vi "SysLog cRIO store messages.vi"(8 "Fehler (in)":errorcluster caption="Fehlerkonstante") -> (0 "Fehler (out)":errorcluster caption="Fehlerkonstante")   [LabVIEW 2020, in "SysLog_cRIO.lvlib"]
doc: "ErrorLogHistory cRIO - Meldungen speichern\nappand to log file - along with BSZ\n\nriw - 11.06.2018"
uses:
  SysLog_cRIO.lvlib
  Allgemein/allgemeine Sub-VIs.lvlib
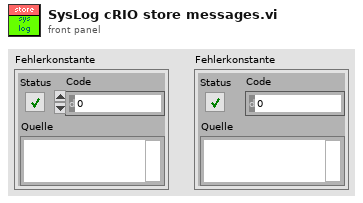
[diagram p1: front panel]
types:
  T1 = enum16{"open", "replace", "create", "open or create", "replace or create", "replace or create with confirmation"}
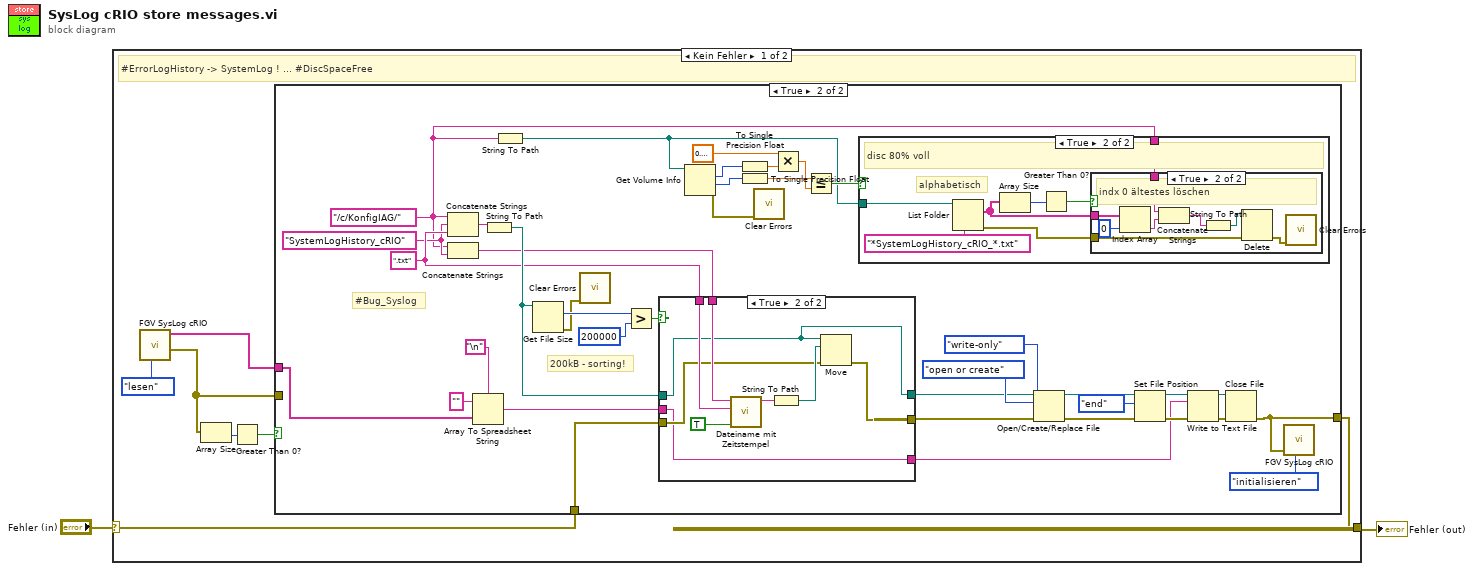
[diagram p0: block diagram]
diagram:
  n1 = case shown="Kein Fehler" "Fehler (in)" {
    selector: "Fehler (in)" -> [w6 w75]
    tunnel: [w5 w75] -> w2
    frame No Error {
      # "#ErrorLogHistory -> SystemLog ! ... #DiscSpaceFree"
      n2 = call "FGV SysLog cRIO.vi"("Aktion"=enum16{"initialisieren", "lesen", "schreiben"}."lesen") -> ("Fehler Array  out"=w3:errorcluster[], "Message out"=w7:string[])  [unwired: 8 in, 1 out]
      n3 = Array Size(array=w3) -> (size(s)=w8:i32)
      n4 = Greater Than 0?(x=w8) -> (x > 0?=w4:bool)
      n5 = case shown="True" w4 {
        tunnel: w7 -> [_ w13]
        tunnel: w3 -> [_ _]
        tunnel: w6 -> [_ w45]
        tunnel: [_ w23] -> w5
        frame False {
        }
        frame True {
          w10 = "/c/KonfigIAG/" ("String")
          w38 = ".txt" ("String")
          w11 = "SystemLogHistory_cRIO" ("String")
          # "#Bug_Syslog"
          # "200kB - sorting!"
          n6 = Concatenate Strings(w10, w11, w38) -> (w40:string)
          n7 = Concatenate Strings(w10, w11) -> (w12:string)
          n8 = Array To Spreadsheet String(delimiter (Tab)="\n", array=w13, 3:"" ("Format-String")) -> (spreadsheet string=w46:string)
          n9 = String To Path(string=w40) -> (path=w39:path)
          n10 = String To Path(string=w10) -> (path=w14:path)
          n11 = Get File Size(file=w39) -> (size (in bytes)=w43:i64, 0:w42:errorcluster)  [unwired: 1 in, 1 out]
          n12 = call <vilib>:"Clear Errors.vi"("error in (no error)"=w42) -> ()  [unwired: 5 in, 2 out]
          n13 = Greater?(x=w43, y=i64 200000) -> (0:w41:bool)
          n14 = case shown="True" w41 {
            tunnel: w46 -> [w64 w66]
            tunnel: w39 -> [w65 w67]
            tunnel: w45 -> [w63 w69]
            tunnel: w12 -> [_ w73]
            tunnel: w38 -> [_ w72]
            tunnel: [w63 w68] -> w27
            tunnel: [w65 w67] -> w28
            tunnel: [w64 w66] -> w26
            frame False {
            }
            frame True {
              n15 = call "Dateiname mit Zeitstempel.vi"("genaue Zeit"=TRUE, "Extension in"=w72, "File Name in"=w73) -> ("File Name"=w71:string)  [unwired: 8 in]
              n16 = String To Path(string=w71) -> (path=w70:path)
              n17 = Move(source path=w67, error in=w69, 10:w70) -> (error out=w68:errorcluster)  [unwired: 2 in, 2 out]
            }
          }
          n18 = Get Volume Info(11:w14) -> (0:w15:errorcluster, 1:w22:i64, 2:w21:i64)  [unwired: 1 in, 3 out]
          n19 = To Single Precision Float(number=w21) -> (single precision float=w17:sgl)
          n20 = To Single Precision Float(number=w22) -> (single precision float=w18:sgl)
          n21 = call <vilib>:"Clear Errors.vi"("error in (no error)"=w15) -> ()  [unwired: 5 in, 2 out]
          n22 = Multiply(x=sgl 0.2, y=w17) -> (x*y=w19:sgl)
          n23 = Less Or Equal?(x=w18, y=w19) -> (x <= y?=w16:bool)
          n24 = case shown="True" w16 {
            tunnel: w14 -> [_ w54]
            tunnel: w10 -> [_ w48]
            frame False {
            }
            frame True {
              # "alphabetisch"
              # "disc 80% voll"
              n25 = List Folder(path=w54, pattern="*SystemLogHistory_cRIO_*.txt" ("Muster")) -> (filenames=w50:string[], error out=w53:errorcluster)  [unwired: 2 in, 2 out]
              n26 = Array Size(array=w50) -> (size(s)=w49:i32)
              n27 = Greater Than 0?(x=w49) -> (x > 0?=w51:bool)
              n28 = case shown="True" w51 {
                tunnel: w53 -> [_ w62]
                tunnel: w50 -> [_ w60]
                tunnel: w48 -> [_ w56]
                frame False {
                }
                frame True {
                  # "indx 0 ältestes löschen"
                  n29 = Index Array(array=w60, index=0 ("Index")) -> (element=w58:string)
                  n30 = Concatenate Strings(w56, w58) -> (w57:string)
                  n31 = String To Path(string=w57) -> (path=w59:path)
                  n32 = Delete(path (use dialog)=w59, error in=w62) -> (error out=w61:errorcluster)  [unwired: 3 in, 2 out]
                  n33 = call <vilib>:"Clear Errors.vi"("error in (no error)"=w61) -> ()  [unwired: 5 in, 2 out]
                }
              }
            }
          }
          n34 = Open/Create/Replace File(file path (use dialog)=w28, error in=w27, operation (0:open)=T1."open or create" ("Operation (0:Öffnen)"), access (0:read/write)=enum16{"read/write", "read-only", "write-only"}."write-only" ("Zugriff (0:Lesen/Schreiben)")) -> (refnum out=w32:refnum<file>, error out=w31:errorcluster)  [unwired: 2 in, 1 out]
          n35 = Set File Position(refnum=w32, from (0:start)=enum16{"start", "end", "current"}."end", error in=w31) -> (refnum out=w30:refnum<file>, error out=w29:errorcluster)  [unwired: 1 in]
          n36 = Write to Text File(file (use dialog)=w30, text=w26, error in=w29) -> (refnum out=w37:refnum<file>, error out=w36:errorcluster)  [unwired: 1 in, 1 out]
          n37 = Close File(refnum=w37, error in=w36) -> (error out=w23:errorcluster)  [unwired: 1 out]
          n38 = call "FGV SysLog cRIO.vi"("Aktion"=enum16{"initialisieren", "lesen", "schreiben"}."initialisieren", "Fehler (in)"=w23) -> ()  [unwired: 7 in, 3 out]
        }
      }
    }
    frame Error {
    }
  }
  "Fehler (out)" <- w2
